vi "instance count allowed.vi"(8 "error in":errorcluster, 11 "configuration in":refnum<class "NISE_CEF_serializable configuration.lvclass">) -> (0 "error out":errorcluster, 2 "instances allowed":i32, 3 "configuration out":refnum<class "NISE_CEF_serializable configuration.lvclass">)   [LabVIEW 2013, in "NISE_CEF_serializable configuration.lvclass"]
doc: "Provides an interface for determining the reentrancy of the runtime class associated with this configuration class. For example, a module which performs processing tasks may allow for unlimited instances (-1) while a component which implements a TCP server may want to limit itself to a smaller number in order to preserve ports. configuration.lvclass provides a value of 0, as no runtime class exists for this configuration."
uses:
  NISE_CEF_serializable configuration.lvclass
  NISE_CEF_TreeControl.lvlib
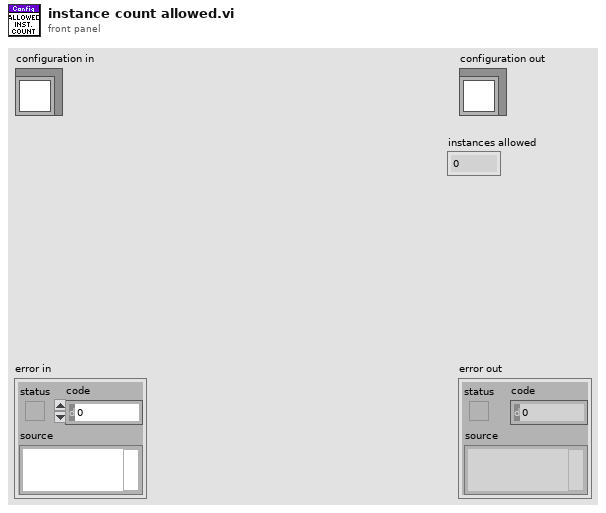
[diagram p1: front panel]
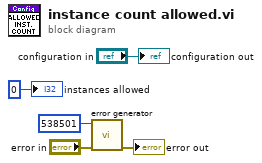
[diagram p0: block diagram]
diagram:
  n1 = call "error generator.vi"("error in"="error in", "error code (0)"=538501) -> ("error out"=→"error out":errorcluster)  [unwired: 7 in]
  "configuration out" <- "configuration in"
  "instances allowed" <- 0 ("instances allowed (-1 = no limit)")
